vi "Register Events.vi"(8 "error in (no error)":errorcluster, 9 "Parameters Table Events":T1, 10 "Channels Table Events":T1, 11 "Event References":T2) -> (0 "error out":errorcluster, 2 "Channel Action":refnum<user-event>, 3 "Event Registration Refnum":refnum<event-registration>)   [LabVIEW 2013, in "control module editor.lvclass"]
uses:
  control module editor.lvclass
  Table API/Table Manager/Table Events.ctl
  Table API/Table Manager/Menu Select.ctl
  Table API/Available Tag Menu/channel action event.ctl
  Table API/Available Tag Menu/dialog output action.ctl
  <vilib>/NI/Tag Bus Module Framework/channel/TBM channel.lvclass
  <vilib>/NI/Tag Bus/tag/tag descriptor.lvclass
  Table API/Table Manager/Call Back Ref Type Def.ctl
  Configuration Editor/Classes/Engine Parent/Engine Parent Editor Node.lvclass
  Configuration Editor/Classes/Module editor node/module editor node.lvclass
  Table API/Table Manager/references.ctl
  <vilib>/NI/Configuration Framework/Node/StopEvent.ctl
  <vilib>/NI/Configuration Framework/Node/RefreshUIEvent.ctl
  <vilib>/NI/Configuration Framework/Node/CacheState.ctl
  <vilib>/NI/Configuration Framework/Node/NodeChangeEvent.ctl
  <vilib>/NI/Configuration Framework/Node/NodeRef.ctl
  <vilib>/NI/Configuration Framework/Node/NISE_CEF_Node.lvclass
  <vilib>/NI/AMC/Message Queue.ctl
  <vilib>/NI/AMC/Message.ctl
  <vilib>/NI/Tools/Keyed Array/KeyedArray.ctl
  <vilib>/NI/Configuration Framework/Node/UserEventRef.ctl
  <vilib>/NI/Configuration Framework/Controls/EventCluster.ctl
  Table API/Table Manager.lvlib
  Table API/Table Manager/Table Manager.lvclass
  <vilib>/NI/Tools/Keyed Array/Tools_KeyedArray.lvlib
  <vilib>/NI/AMC/AMC.lvlib
  <vilib>/NI/Configuration Framework/NISE_CEF_TreeControl.lvlib
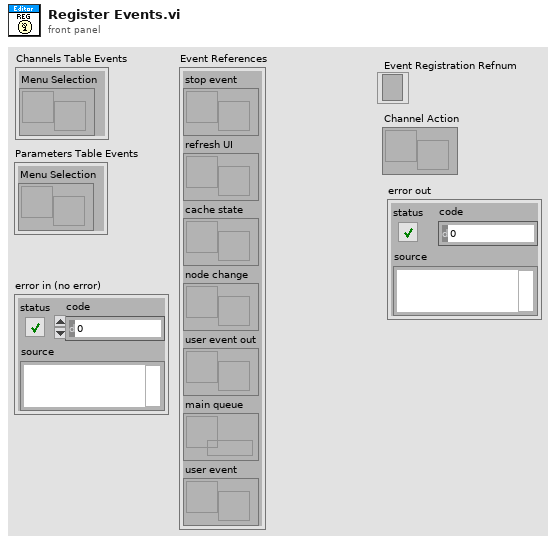
[diagram p1: front panel]
types:
  T1 = typedef "Table Manager.lvlib/Table Manager.lvclass/Table Events.ctl" = cluster{"Menu Selection":refnum<user-event>}
  T2 = typedef "Table Manager.lvlib/Table Manager.lvclass/references.ctl" = cluster{"stop event":T3, "refresh UI":T4, "cache state":T5, "node change":T6, "user event out":refnum<user-event>, "main queue":T7, "user event":T8}
  T3 = typedef "NISE_CEF_Node.lvclass/StopEvent.ctl" = refnum<user-event>
  T4 = typedef "NISE_CEF_Node.lvclass/RefreshUIEvent.ctl" = refnum<user-event>
  T5 = typedef "NISE_CEF_Node.lvclass/CacheState.ctl" = refnum<user-event>
  T6 = typedef "NISE_CEF_Node.lvclass/NodeChangeEvent.ctl" = refnum<user-event>
  T7 = typedef "AMC.lvlib/Message Queue.ctl" = refnum<queue>
  T8 = typedef "NISE_CEF_Node.lvclass/UserEventRef.ctl" = refnum<user-event>
  T9 = typedef "Table Manager.lvlib/channel action event.ctl" = cluster{"action":T10, "channel":refnum<class "TBM channel.lvclass">, "selected tag":refnum<class "tag descriptor.lvclass">, "Call Back VI":T11}
  T10 = typedef "Table Manager.lvlib/dialog output action.ctl" = enum16{"Tag Created", "Tag Selected", "Set Default", "disconnect"}
  T11 = typedef "Table Manager.lvlib/Table Manager.lvclass/Call Back Ref Type Def.ctl" = refnum<vi>
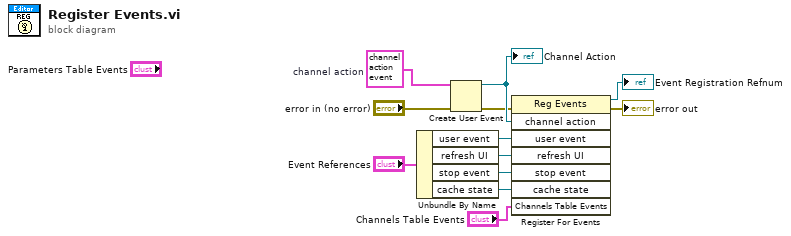
[diagram p0: block diagram]
diagram:
  w5 = T9 {"action"=enum."Tag Created", "channel"=refnum, "selected tag"=refnum, "Call Back VI"=refnum}  # channel action
  n1 = Unbundle By Name("Event References") -> ("user event"=w11:T8, "refresh UI"=w7:T4, "stop event"=w9:T3, "cache state"=w10:T5)
  n2 = Create User Event(user event datatype=w5, error in="error in (no error)") -> (user event=w8:refnum<user-event>, error out=w4:errorcluster)
  "Channel Action" <- w8
  n3 = register-events(error in=w4, w8, w11, w7, w9, w10, "Channels Table Events") -> (reference out=→"Event Registration Refnum":refnum<event-registration>, error out=→"error out":errorcluster)  [unwired: 1 in]
